vi "Notify.vi"(0 "reference in":refnum<class "Mediator.lvclass">, 2 "Sender":string, 5 "error in (no error)":errorcluster, 10 "Message":string) -> (14 "reference out":refnum<class "Mediator.lvclass">, 19 "error out":errorcluster)   [LabVIEW 2013, in "Mediator.lvclass"]
uses:
  Mediator.lvclass
  Colleague_class/Colleague.lvclass
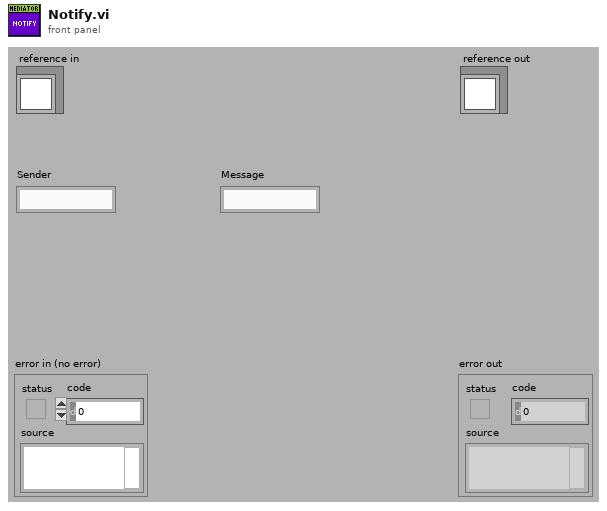
[diagram p1: front panel]
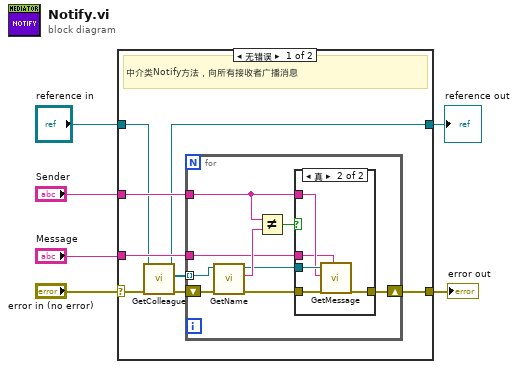
[diagram p0: block diagram]
diagram:
  n1 = case shown="无错误" "error in (no error)" {
    selector: "error in (no error)" -> [w10 w31]
    tunnel: [w9 w31] -> w5
    tunnel: [w7 w30] -> w3
    tunnel: "reference in" -> [w8 w30]
    tunnel: "Sender" -> [w12 _]
    tunnel: "Message" -> [w11 _]
    frame No Error {
      # "中介类Notify方法，向所有接收者广播消息"
      n2 = call-dynamic "GetColleague.vi"("error in (no error)"=w10, "reference in"=w8) -> ("error out"=w13:errorcluster, "Colleague"=w14:refnum<class "Colleague.lvclass">[], "reference out"=w7:refnum<class "Mediator.lvclass">)  [unwired: 7 in]
      n3 = for {
        tunnel: w14 -> [w23] mode=indexing
        shift-right: [w16] -> w9
        shift-left: w13 -> [w22]
        tunnel: w12 -> [w18]
        tunnel: w11 -> [w17]
        n4 = call "GetName.vi"("error in (no error)"=w22, "reference in"=w23) -> ("error out"=w15:errorcluster, "Name"=w21:string, "reference out"=w19:refnum<class "Colleague.lvclass">)  [unwired: 7 in]
        n5 = Not Equal?(x=w18, y=w21) -> (x != y?=w20:bool)
        n6 = case shown="真" w20 {
          tunnel: w19 -> [_ w29]
          tunnel: w18 -> [_ w28]
          tunnel: w17 -> [_ w27]
          tunnel: [w24 w26] -> w16
          tunnel: w15 -> [w24 w25]
          frame False {
          }
          frame True {
            n7 = call-dynamic "GetMessage.vi"("reference in"=w29, "Sender"=w28, "error in (no error)"=w25, "Message"=w27) -> ("error out"=w26:errorcluster)  [unwired: 14 in, 1 out]
          }
        }
      }
    }
    frame Error {
    }
  }
  "error out" <- w5
  "reference out" <- w3
